vi "Neg Binomial Inverse CDF.vi"(9 "p":dbl=0.02, 10 "x":dbl=1.0, 11 "cdf(y)":dbl=0.5) -> (0 "error":i32, 3 "y":i32)   [LabVIEW 2018, in "NI_Gmath.lvlib"]
doc: "Computes the discrete inverse cumulative distribution function (CDF), or the value <B>x</B> such that the probability that the random variate X, where X describes the selected distribution type, takes on a value less than or equal to it is <B>cdf(x)</B>. You must manually select the polymorphic instance to use."
uses:
  NI_Gmath.lvlib
panel:
  # "Negative Binomial Inverse CDF"
  # "failures"
  # "successes"
  # "probability"
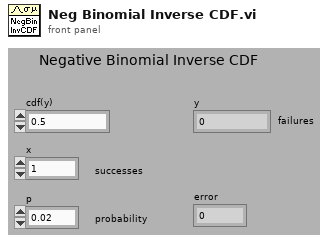
[diagram p1: front panel]
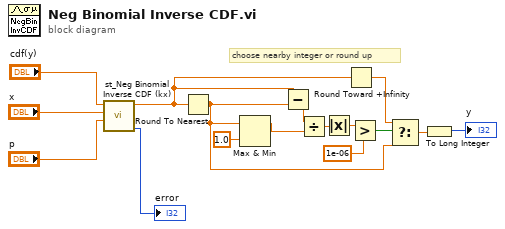
[diagram p0: block diagram]
diagram:
  # "choose nearby integer or round up"
  n1 = call "st_Neg Binomial Inverse CDF (kx).vi"("p"="p", "x"="x", "cdf(y)"="cdf(y)") -> ("error"=→"error":i32, "y"=w4:dbl)  [unwired: 7 in]
  n2 = Round To Nearest(number=w4) -> (nearest integer value=w2:dbl)
  n3 = Max & Min(x=w2, y=1.0) -> (max(x,y)=w1:dbl)  [unwired: 1 out]
  n4 = Subtract(x=w4, y=w2) -> (x-y=w15:dbl)
  n5 = Divide(x=w15, y=w1) -> (x/y=w13:dbl)
  n6 = Absolute Value(x=w13) -> (abs(x)=w14:dbl)
  n7 = Round Toward +Infinity(x=w4) -> (ceil(x): smallest int >= x=w10:dbl)
  n8 = Greater?(x=w14, y=1e-06) -> (0:w11:bool)
  n9 = Select(t=w10, s=w11, f=w2) -> (s? t:f=w16:dbl)
  n10 = To Long Integer(number=w16) -> (32bit integer=→"y":i32)
